vi "num2lett.vi"(11 "Number":i32) -> (3 "Letter":string)   [LabVIEW 2019]
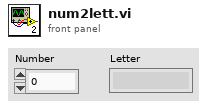
[diagram p1: front panel]
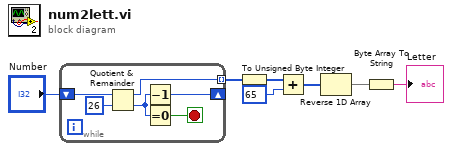
[diagram p0: block diagram]
diagram:
  n1 = while {
    tunnel: [w12] -> w1 mode=indexing
    shift-right: [w8] -> _
    shift-left: "Number" -> [w13]
    stop <- w11 stop-if-true
    n2 = Quotient & Remainder(x=w13, y=26) -> (x-y*floor(x/y)=w12:i32, floor(x/y)=w10:i32)
    n3 = Decrement(x=w10) -> (x-1=w8:i32)
    n4 = Equal To 0?(x=w10) -> (x = 0?=w11:bool)
  }
  n5 = To Unsigned Byte Integer(number=w1) -> (unsigned 8bit integer=w6:u8[])
  n6 = Add(x=w6, y=u8 65) -> (x+y=w4:u8[])
  n7 = Reverse 1D Array(array=w4) -> (reversed array=w2:u8[])
  n8 = Byte Array To String(unsigned byte array=w2) -> (string=→"Letter":string)
